vi "Read previous.vi"(11 "Node in":refnum<class "Node.lvclass">) -> (2 "previous":refnum<data-value>, 3 "Node out":refnum<class "Node.lvclass">)   [LabVIEW 2023, in "d20.lvlib" / "Node.lvclass"]
uses:
  Node.lvclass
  INode/INode.lvclass
  Node.lvclass/Node.ctl
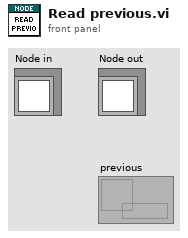
[diagram p1: front panel]
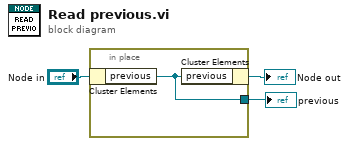
[diagram p0: block diagram]
diagram:
  n1 = in-place {
    in-place-border: [w4] -> w3
    n2 = in-place-cluster #1("Node in") -> ("previous"=w4:refnum<data-value>)
    n3 = in-place-cluster #1("previous"=w4) -> (→"Node out":refnum<class "Node.lvclass">)
  }
  "previous" <- w3
